vi "DOWNSAMPLING - Type.vi"(8 "error in (no error)":errorcluster, 11 "Downsampling Type":T1) -> (0 "error out":errorcluster, 3 "DOWNSAMPLING_TYPE_VALUE":i32)   [LabVIEW 2018]
doc: "<b>Downsampling type, switch between binning and skipping, to be used with the PRM.DOWNSAMPLING_TYPE function parameter.</b>\nDOWNSAMPLING_TYPE.BINNING : Binned type for higher sensitivity.\nDOWNSAMPLING_TYPE.SKIPPING : Skipped type for higher framerates."
uses:
  DOWNSAMPLING_TYPE.ctl
  D:/codes labview/VisionLibrariesXimea/xiLib/xiLIB_64bit/xiLIB/xiCamLib/API/x64/xiApi.NETX64.dll
  API/x64/xiApi.NETX64.dll
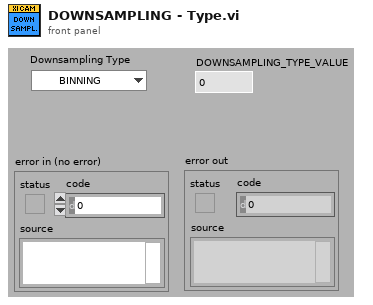
[diagram p1: front panel]
types:
  T1 = typedef "DOWNSAMPLING_TYPE.ctl" = enum16{"BINNING", "SKIPPING"}
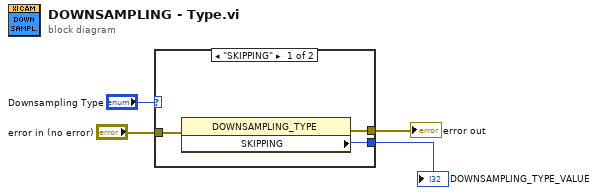
[diagram p0: block diagram]
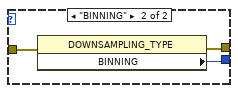
[diagram p2: hidden frame]
diagram:
  n1 = case shown="\"SKIPPING\"" "Downsampling Type" {
    tunnel: "error in (no error)" -> [w7 w10]
    tunnel: [w6 w9] -> w2
    tunnel: [w5 w8] -> w1
    frame "SKIPPING" {
      n2 = property class="DOWNSAMPLING_TYPE"(error in=w7) -> (error out=w6:errorcluster, "SKIPPING"=w5:i32)  [unwired: 1 in, 1 out]
    }
    frame "BINNING" {
      n3 = property class="DOWNSAMPLING_TYPE"(error in=w10) -> (error out=w9:errorcluster, "BINNING"=w8:i32)  [unwired: 1 in, 1 out]
    }
  }
  "error out" <- w2
  "DOWNSAMPLING_TYPE_VALUE" <- w1
